vi "PFI-28000-Chan-Bridge_Set Filter Type.vi"(8 "error in (no error)":errorcluster, 10 "Filter Type":T1, 11 "PFI-28000-Chan-Bridge in":refnum<class "PFI-28000-Chan-Bridge.lvclass">) -> (0 "error out":errorcluster, 3 "PFI-28000-Chan-Bridge out":refnum<class "PFI-28000-Chan-Bridge.lvclass">)   [LabVIEW 2017, in "PFI-28000-Chan-Bridge.lvclass"]
uses:
  PFI-28000-Chan-Bridge.lvclass
  C:/wc/07143 Precision Filters 28000 Support/Driver/source/Channel/PFI-28000-Channel.lvclass
  PFI-28000-Chan-Bridge-Filter Type.ctl
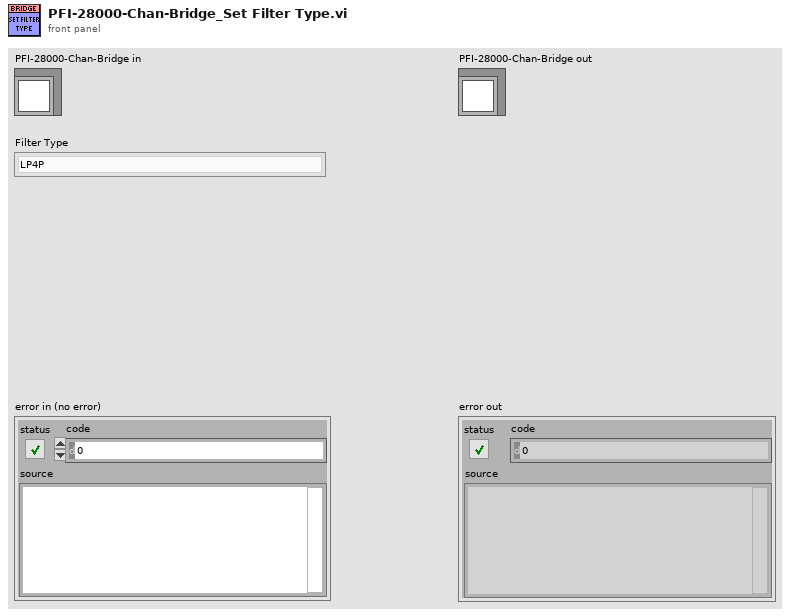
[diagram p1: front panel]
types:
  T1 = typedef "PFI-28000-Chan-Bridge.lvclass/PFI-28000-Chan-Bridge-Filter Type.ctl" = enum8{"LP4P", "LP4F"}
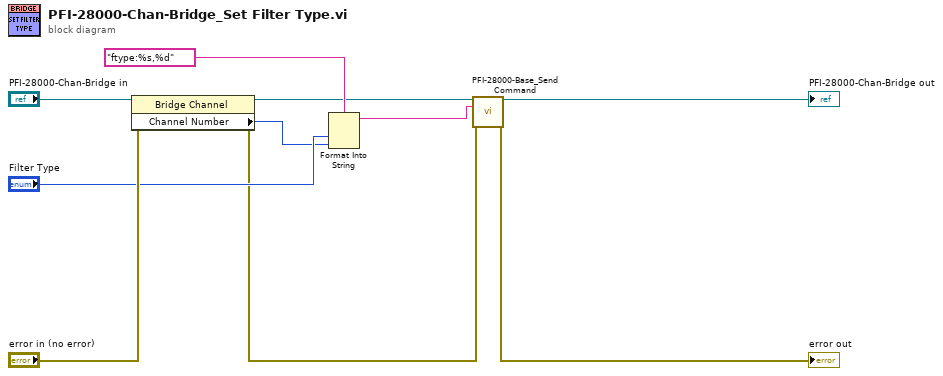
[diagram p0: block diagram]
diagram:
  n1 = property class="Bridge Channel"(reference="PFI-28000-Chan-Bridge in", error in="error in (no error)") -> (reference out=w4:refnum<class "PFI-28000-Chan-Bridge.lvclass">, error out=w2:errorcluster, "Channel Number"=w6:i32)
  n2 = Format Into String(format string="ftype:%s,%d" ("empty string"), "Filter Type", w6) -> (resulting string=w5:string)  [unwired: 2 in, 1 out]
  n3 = call-dynamic "PFI-28000-Base_Send Command.vi"("PFI-28000-Base in"=w4, "Command"=w5, "error in (no error)"=w2) -> ("PFI-28000-Base out"=→"PFI-28000-Chan-Bridge out":refnum<class "PFI-28000-Chan-Bridge.lvclass">, "error out"=→"error out":errorcluster)  [unwired: 11 in]
